vi "Configure RJDJ Extraction Measurement.vi"(0 "VISA resource name":refnum<visa-resource-name>, 1 "Enable RJDJ Measurement (Enable)":bool, 2 "BER Level (6: 1E-12)":i32(ring) items=["1E-6", "1E-7", "1E-8", "1E-9", "1E-10", "1E-11", "1E-12", "1E-13", "1E-14", "1E-15", "1E-16", "1E-17", "1E-18"], 5 "Source (1: Channel 1)":i32(ring) items=["Channel 1", "Channel 2", "Channel 3", "Channel 4", "Function 1", "Function 2", "Function 3", "Function 4", "Memory 1", "Memory 2", "Memory 3", "Memory 4"], 7 "Bandwidth (0: Narrow)":i32(ring) items=["Narrow (Pink)", "Wide (White)"], 9 "Edge (2: Both)":i32(ring) items=["Rising", "Falling ", "Both"], 11 "error in (no error)":errorcluster, 12 "Interpolation Mode (0: None)":i32(ring) items=["None", "Linear"], 13 "Measurement Units (0: Second)":i32(ring) items=["Second", "Unit Interval"], 14 "Pattern Length":T1 {"Pattern Length Type (0: Periodic)" items=["Periodic", "Periodic (Number of Bits)", "Arbitrary"]}) -> (4 "VISA resource name out":refnum<visa-resource-name>, 15 "error out":errorcluster)   [LabVIEW 2009, in "Agilent 8000 Series.lvlib"]
doc: "Configures the RJDJ Extraction Measurement and its parameters. Calling this VI enables the RJDJ extraction measurement on the selected channel.\n\n<b>Note: </b>\n\nThis VI is only for the Agilent 80000 Series. It does not support the Agilent 8000 Series."
uses:
  Agilent 8000 Series.lvlib
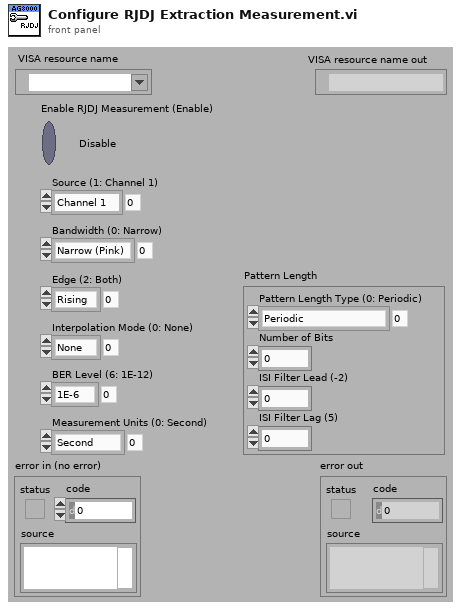
[diagram p1: front panel]
types:
  T1 = cluster{"ISI Filter Lead (-2)":dbl, "ISI Filter Lag (5)":dbl, "Pattern Length Type (0: Periodic)":i32, "Number of Bits":u32}
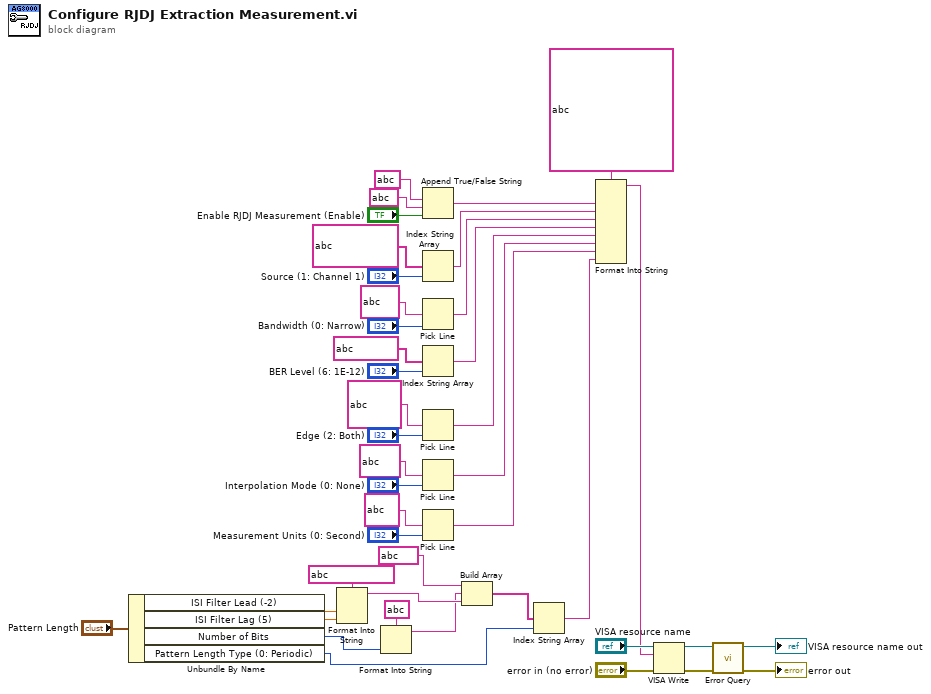
[diagram p0: block diagram]
diagram:
  n1 = Unbundle By Name("Pattern Length") -> ("ISI Filter Lead (-2)"=w26:dbl, "ISI Filter Lag (5)"=w25:dbl, "Number of Bits"=w8:u32, "Pattern Length Type (0: Periodic)"=w5:i32)
  n2 = Format Into String(format string=string ?, w26, w25) -> (resulting string=w2:string)  [unwired: 2 in, 1 out]
  n3 = Format Into String(format string=string ?, w8) -> (resulting string=w1:string)  [unwired: 2 in, 1 out]
  n4 = Append True/False String(1:"Enable RJDJ Measurement (Enable)", 2:string ? ("false string"), 3:string ? ("true string")) -> (0:w22:string)  [unwired: 1 in]
  n5 = Index String Array(1:"Source (1: Channel 1)", 2:string[] ?) -> (0:w20:string)  [unwired: 1 in]
  n6 = Pick Line(multi-line string=string ?, line index="Bandwidth (0: Narrow)") -> (output string=w19:string)  [unwired: 1 in]
  n7 = Index String Array(1:"BER Level (6: 1E-12)", 2:string[] ?) -> (0:w21:string)  [unwired: 1 in]
  n8 = Pick Line(multi-line string=string ?, line index="Edge (2: Both)") -> (output string=w18:string)  [unwired: 1 in]
  n9 = Pick Line(multi-line string=string ?, line index="Interpolation Mode (0: None)") -> (output string=w17:string)  [unwired: 1 in]
  n10 = Pick Line(multi-line string=string ?, line index="Measurement Units (0: Second)") -> (output string=w16:string)  [unwired: 1 in]
  n11 = Build Array(string ? ("format string"), w1, w2) -> (w4:string[])
  n12 = Index String Array(1:w5, 2:w4) -> (0:w3:string)  [unwired: 1 in]
  n13 = Format Into String(format string=string ?, w22, w20, w19, w21, w18, w17, w16, w3) -> (resulting string=w9:string)  [unwired: 2 in, 1 out]
  n14 = VISA Write(VISA resource name="VISA resource name", write buffer=w9, error in (no error)="error in (no error)") -> (VISA resource name out=w14:refnum<visa-resource-name>, error out=w11:errorcluster)  [unwired: 1 out]
  n15 = call "Error Query.vi"("error in (no error)"=w11, "VISA resource name"=w14) -> ("error out"=→"error out":errorcluster, "VISA resource name out"=→"VISA resource name out":refnum<visa-resource-name>)  [unwired: 6 in, 2 out]
